vi "Guassian_2D.vi"(3 "output control":T1, 4 "data":T2, 5 "X":dbl[](array[numeric]), 6 "a":dbl[](array[numeric])) -> (0 "error out":errorcluster, 1 "f'(X,a)":dbl[][](array[numeric]), 2 "f(X,a)":dbl[](array[numeric]))   [LabVIEW 2014]
doc: "This template is the starting point for creating a model function to be passed to the Nonlinear Curve Fit.vi."
uses:
  <vilib>/gmath/NumericalOptimization/objective function data.ctl
  <vilib>/gmath/NumericalOptimization/LM_output select.ctl
  <vilib>/gmath/NI_Gmath.lvlib
panel:
  # "Amp\nXo\nYo\nWx\nWy\nOffset"
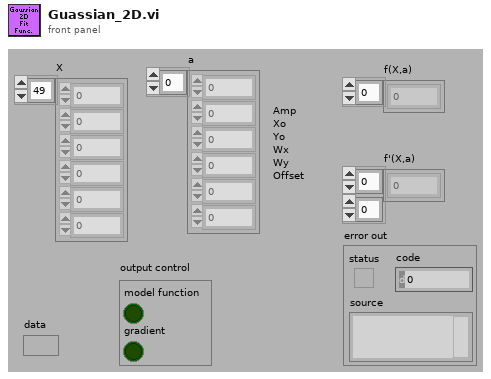
[diagram p1: front panel]
types:
  T1 = typedef "NI_Gmath.lvlib/LM_output select.ctl" = cluster{"model function":bool, "gradient":bool}
  T2 = typedef "NI_Gmath.lvlib/objective function data.ctl" = variant
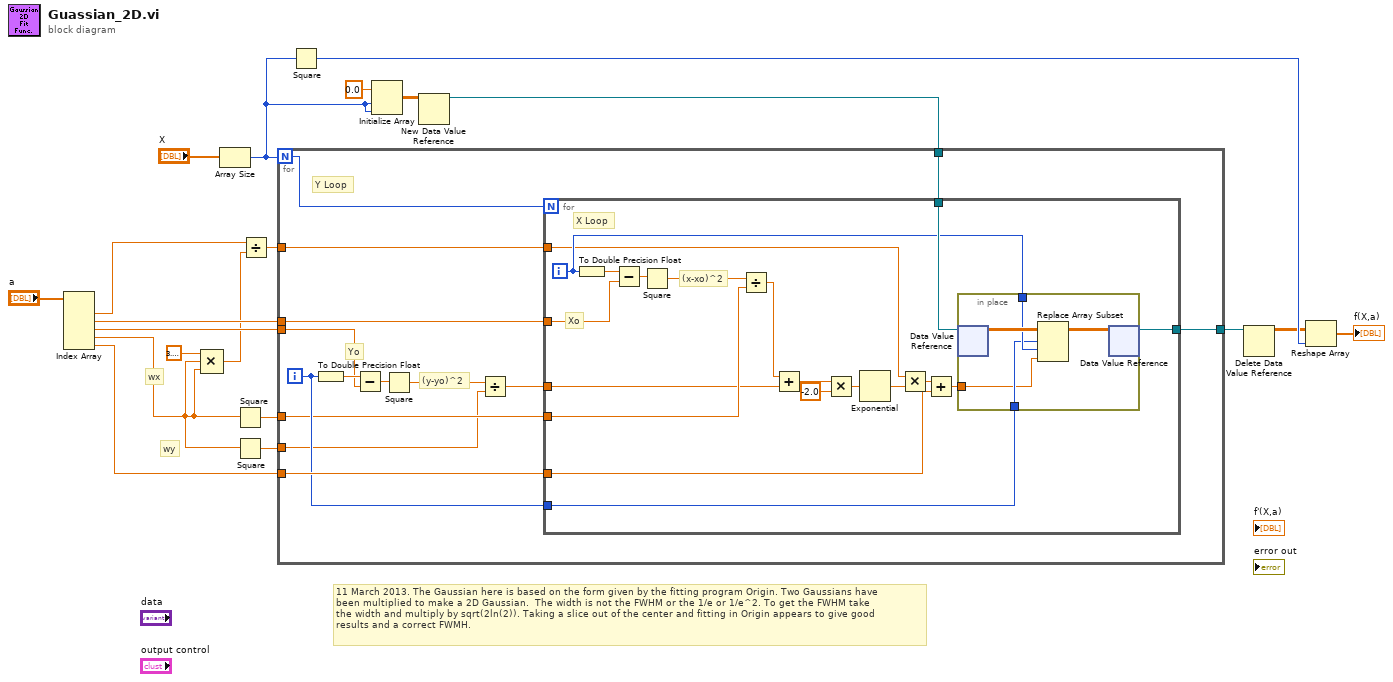
[diagram p0: block diagram]
diagram:
  # "11 March 2013. The Gaussian here is based on the form given by the fitting program Origin. Two Gaussians have\nbeen multiplied to make a 2D Gaussian.  The width is not the FWHM or the 1/e or 1/e^2. To get the FWHM take\nthe width and multiply by sqrt(2ln(2)). Taking a slice out of the center and fitting in Origin appears to give good\nresults and a correct FWMH."
  # "wy"
  # "wx"
  n1 = Index Array(array="a") -> (element #1=w6:dbl, element #2=w18:dbl, element #3=w17:dbl, element #4=w2:dbl, element #5=w1:dbl)  [unwired: 5 in]
  n2 = Compound Arithmetic op=MULTIPLY(3.141592653589793, w2, w2) -> (w5:dbl)
  n3 = Array Size(array="X") -> (size(s)=w11:i32)
  n4 = Square(x=w2) -> (x^2=w9:dbl)
  n5 = Square(x=w2) -> (x^2=w8:dbl)
  n6 = Divide(x=w6, y=w5) -> (x/y=w4:dbl)
  n7 = Square(x=w11) -> (x^2=w10:i32)
  n8 = Initialize Array(0.0 ("element"), w11, w11) -> (w15:dbl[][])
  n9 = New Data Value Reference(data value=w15) -> (data value reference=w14:refnum<data-value>)  [unwired: 1 in, 1 out]
  n10 = for {
    N: w11 -> [w34]
    tunnel: w18 -> [w33]
    tunnel: w17 -> [w30]
    tunnel: w1 -> [w32]
    tunnel: w14 -> [w28]
    tunnel: [w26] -> w13
    tunnel: w9 -> [w25]
    tunnel: w8 -> [w23]
    tunnel: w4 -> [w21]
    i -> [w27]
    # "(y-yo)^2"
    # "Yo"
    # "Y Loop"
    n11 = To Double Precision Float(number=w27) -> (double precision float=w31:dbl)
    n12 = Subtract(x=w31, y=w30) -> (x-y=w29:dbl)
    n13 = Square(x=w29) -> (x^2=w24:dbl)
    n14 = Divide(x=w24, y=w23) -> (x/y=w22:dbl)
    n15 = for {
      N: w34 -> [_]
      tunnel: w33 -> [w52]
      tunnel: w32 -> [w50]
      tunnel: w28 -> [w49]
      tunnel: w27 -> [w47]
      tunnel: [w45] -> w26
      tunnel: w25 -> [w43]
      tunnel: w22 -> [w42]
      tunnel: w21 -> [w35]
      i -> [w48]
      # "Xo"
      # "(x-xo)^2"
      # "X Loop"
      n16 = To Double Precision Float(number=w48) -> (double precision float=w53:dbl)
      n17 = Subtract(x=w53, y=w52) -> (x-y=w51:dbl)
      n18 = Square(x=w51) -> (x^2=w44:dbl)
      n19 = Divide(x=w44, y=w43) -> (x/y=w41:dbl)
      n20 = Add(x=w41, y=w42) -> (x+y=w40:dbl)
      n21 = Multiply(x=w40, y=-2.0) -> (x*y=w38:dbl)
      n22 = Exponential(1:w38) -> (0:w37:dbl)
      n23 = Multiply(x=w35, y=w37) -> (x*y=w36:dbl)
      n24 = Add(x=w36, y=w50) -> (x+y=w46:dbl)
      n25 = in-place {
        in-place-border: w48 -> [w56]
        in-place-border: w47 -> [w55]
        in-place-border: w46 -> [w54]
        n26 = in-place-dvr #1(w49) -> (w58:dbl[][])  [unwired: 1 out]
        n27 = Replace Array Subset(array=w58, new element=w54, index (row)=w55, index (col)=w56) -> (w57:dbl[][])
        n28 = in-place-dvr #1(w57) -> (w45:refnum<data-value>)  [unwired: 1 out]
      }
    }
  }
  n29 = Delete Data Value Reference(data value reference=w13) -> (data value=w3:dbl[][])  [unwired: 1 in, 1 out]
  n30 = Reshape Array(w3, w10) -> (→"f(X,a)":dbl[])
